vi "Set delay.vi"(7 "[x]":T1, 8 "error in (no error)":errorcluster, 10 "Delay (min)":dbl[](array[numeric]), 11 "Serial Port in":refnum<visa-resource-name>) -> (0 "error out":errorcluster, 3 "Serial Port out":refnum<visa-resource-name>)   [LabVIEW 2016, in "Chemyx_Syringe_Pump_driver.lvlib"]
doc: "Sets a delay before start of the syringe pump.\n\nDelay is a double float. Units are minutes. \n\nIf you want the system to run at a certain point in your setup\n(i.e. after, 1030\nseconds, 1, 5, 10 minutes, etc.) you may set a time delay for appropriate time for pump to begin\nrun."
uses:
  Chemyx_Syringe_Pump_driver.lvlib
  _private/Control/Control Mode.ctl
panel:
  # "Sets the delay of the pump syringe"
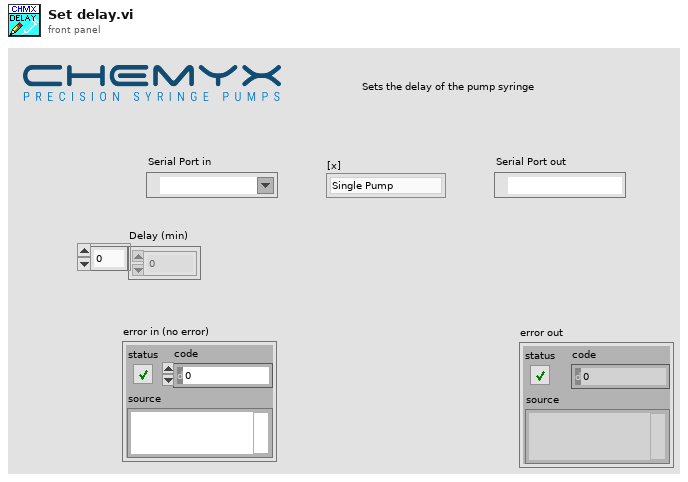
[diagram p1: front panel]
types:
  T1 = typedef "Chemyx_Syringe_Pump_driver.lvlib/Control Mode.ctl" = enum16{"Single Pump", "Pump Chanel 1", "Pump Channel 2", "Cycle Mode"}
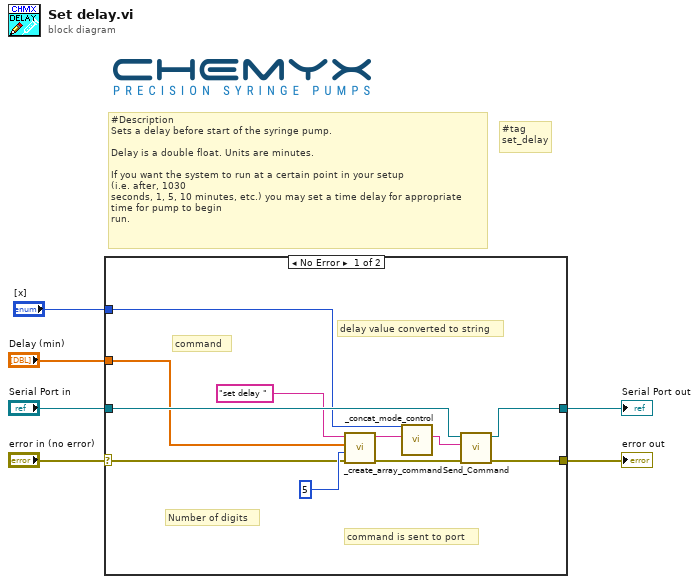
[diagram p0: block diagram]
diagram:
  # "#tag\nset_delay"
  # "#Description\nSets a delay before start of the syringe pump.\n\nDelay is a double float. Units are minutes. \n\nIf you want the system to run at a certain point in your setup\n(i.e. after, 1030\nseconds, 1, 5, 10 minutes, etc.) you may set a time delay for appropriate time for pump to begin\nrun."
  n1 = case shown="No Error" "error in (no error)" {
    selector: "error in (no error)" -> [w10 w19]
    tunnel: "Serial Port in" -> [w17 w18]
    tunnel: [w16 w19] -> w4
    tunnel: [w15 w18] -> w3
    tunnel: "Delay (min)" -> [w12 _]
    tunnel: "[x]" -> [w7 _]
    frame No Error {
      # "Number of digits"
      # "command is sent to port"
      # "delay value converted to string"
      # "command"
      n2 = call "_create_array_command.vi"("error in"=w10, "precision (1)"=i16 5 ("precision (6)"), "array"=w12, "Command in"="set delay ") -> ("error out"=w11:errorcluster, "Command out"=w9:string)  [unwired: 6 in]
      n3 = call "_concat_mode_control.vi"("write buffer"=w9, "[x]"=w7) -> ("write buffer out"=w8:string)  [unwired: 9 in]
      n4 = call "Send_Command.vi"("error in (no error)"=w11, "write buffer"=w8, "Serial Port in"=w17) -> ("error out"=w16:errorcluster, "VISA Refnum out"=w15:refnum<visa-resource-name>)  [unwired: 6 in, 1 out]
    }
    frame Error {
    }
  }
  "error out" <- w4
  "Serial Port out" <- w3
